vi "稳定条件判断.vi"(11 "变异系数":dbl) -> (3 "布尔":bool)   [LabVIEW 2016, in "斯坦道多参数.lvlib"]
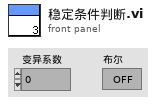
[diagram p1: front panel]
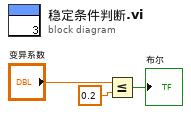
[diagram p0: block diagram]
diagram:
  n1 = Less Or Equal?(x="变异系数", y=0.2) -> (x <= y?=→"布尔":bool)
